vi "Add Tags.vi"(9 "Tag Values":string[](array[string]), 10 "Tags":string[](array[string]), 11 "Packet in":string) -> (3 "Packet out":string)   [LabVIEW 2011, in "StatD Interface.lvclass"]
doc: "Adds tags to the end of the packet if any are specified."
uses:
  StatD Interface.lvclass
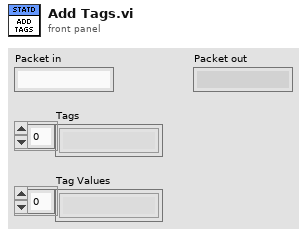
[diagram p1: front panel]
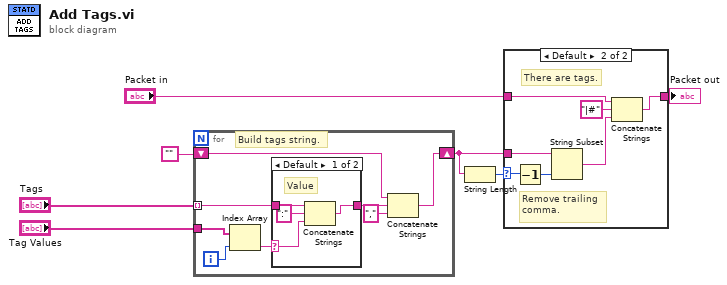
[diagram p0: block diagram]
diagram:
  n1 = for {
    tunnel: "Tags" -> [w12] mode=indexing
    tunnel: "Tag Values" -> [w14]
    shift-right: [w10] -> w4
    shift-left: "" -> [w11]
    i -> [w15]
    # "Build tags string."
    n2 = Index Array(array=w14, index=w15) -> (element=w13:string)
    n3 = case shown="Default" w13 {
      selector: w13 -> [w17 _]
      tunnel: w12 -> [w18 w20]
      tunnel: [w19 w20] -> w9
      frame Default {
        # "Value"
        n4 = Concatenate Strings(w18, ":" ("string"), w17) -> (w19:string)
      }
      frame "" {
        # "No Value"
      }
    }
    n5 = Concatenate Strings(w11, w9, "," ("string")) -> (w10:string)
  }
  n6 = String Length(string=w4) -> (length=w5:i32)
  n7 = case shown="Default" w5 {
    selector: w5 -> [_ w26]
    tunnel: w4 -> [_ w27]
    tunnel: [w21 w25] -> w6
    tunnel: "Packet in" -> [w21 w24]
    frame 0 {
      # "No Tags"
    }
    frame Default {
      # "There are tags."
      # "Remove trailing\ncomma."
      n8 = Decrement(x=w26) -> (x-1=w28:i32)
      n9 = String Subset(string=w27, length (rest)=w28) -> (substring=w22:string)  [unwired: 1 in]
      n10 = Concatenate Strings(w24, "|#" ("string"), w22) -> (w25:string)
    }
  }
  "Packet out" <- w6
